vi "LOGlog.vi"(7 "Level":u8, 8 "Error In":errorcluster, 10 "Message":T1, 11 "Listeners In":refnum<queue>[](array[refnum])) -> (0 "Error Out":errorcluster, 3 "Listeners Out":refnum<queue>[](array[refnum]))   [LabVIEW 2025]
uses:
  LOGstatement.ctl
  <vilib>/Field R&D Services/Logger/Type Definitions/Tag.ctl
  <vilib>/Field R&D Services/Logger/Field_RnD_Services_Logger_Toolkit.lvlib
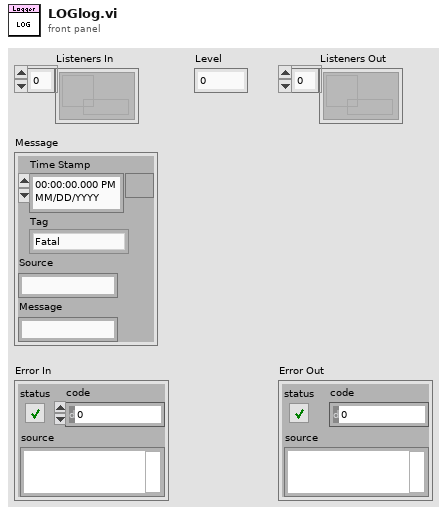
[diagram p1: front panel]
types:
  T1 = typedef "Field_RnD_Services_Logger_Toolkit.lvlib/LOGstatement.ctl" = cluster{"Time Stamp":timestamp, "Tag":T2, "Source":string, "Message":string}
  T2 = typedef "Field_RnD_Services_Logger_Toolkit.lvlib/Tag.ctl" = enum16{"Fatal", "Error", "Warn", "Info", "Debug", "Trace"}
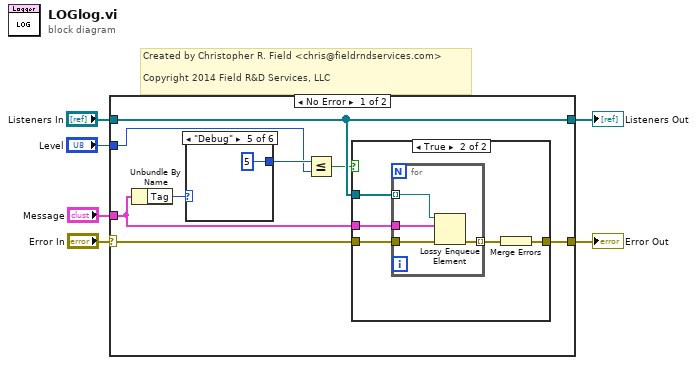
[diagram p0: block diagram]
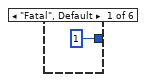
[diagram p3: hidden frame]
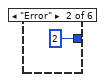
[diagram p4: hidden frame]
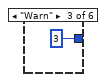
[diagram p5: hidden frame]
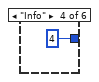
[diagram p6: hidden frame]
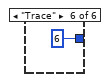
[diagram p7: hidden frame]
diagram:
  # "Created by Christopher R. Field <chris@fieldrndservices.com>\n\nCopyright 2014 Field R&D Services, LLC"
  n1 = case shown="No Error" "Error In" {
    selector: "Error In" -> [w12 w31]
    tunnel: "Message" -> [w11 _]
    tunnel: [w14 w31] -> w5
    tunnel: "Listeners In" -> [w13 w32]
    tunnel: [w13 w32] -> w3
    tunnel: "Level" -> [w7 _]
    frame No Error {
      n2 = Unbundle By Name(w11) -> ("Tag"=w10:T2)
      n3 = case shown="\"Debug\"" w10 {
        tunnel: [1 2 3 4 5 6] -> w8
        frame "Fatal", Default {
        }
        frame "Error" {
        }
        frame "Warn" {
        }
        frame "Info" {
        }
        frame "Debug" {
        }
        frame "Trace" {
        }
      }
      n4 = Less Or Equal?(x=w8, y=w7) -> (x <= y?=w9:bool)
      n5 = case shown="True" w9 {
        tunnel: [w15 w16] -> w14
        tunnel: w13 -> [_ w20]
        tunnel: w12 -> [w15 w19]
        tunnel: w11 -> [_ w18]
        frame False {
        }
        frame True {
          n6 = for {
            tunnel: w20 -> [w24] mode=indexing
            tunnel: w18 -> [w22]
            tunnel: w19 -> [w23]
            tunnel: [w21] -> w17 mode=indexing
            n7 = Lossy Enqueue Element(queue=w24, element=w22, error in (no error)=w23) -> (error out=w21:errorcluster)  [unwired: 3 out]
          }
          n8 = Merge Errors(w17) -> (w16:errorcluster)
        }
      }
    }
    frame Error {
    }
  }
  "Error Out" <- w5
  "Listeners Out" <- w3
